vi "From XML.vi"(8 "error in (no error)":errorcluster, 10 "XML String":string, 11 "TOC in":refnum<class "TOC.lvclass">) -> (0 "error out":errorcluster, 3 "TOC out":refnum<class "TOC.lvclass">)   [LabVIEW 2015, in "TOC.lvclass"]
uses:
  TOC.lvclass
  <vilib>/xml/Load XML String.vi
  <vilib>/xml/NI_XML.lvlib
  <resource>/objmgr/DOMUserDefRef.rc
panel:
  out "Node Name":string
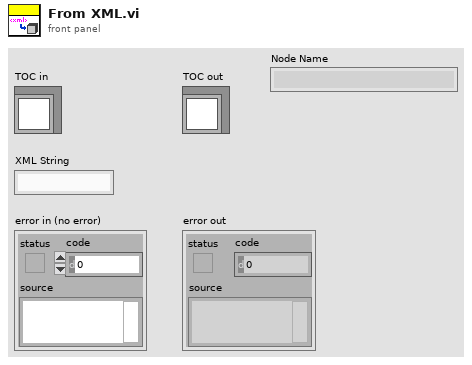
[diagram p1: front panel]
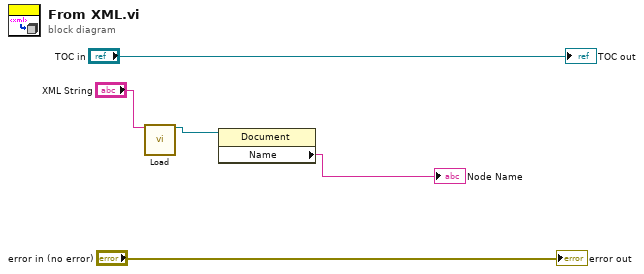
[diagram p0: block diagram]
diagram:
  n1 = call-poly <vilib>:"Load.vi"("XML string"="XML String") -> ("DOM document out"=w2:refnum<k20>)  [unwired: 12 in, 2 out]
  n2 = property class="Document"(reference=w2) -> ("Name"=→"Node Name":string)  [unwired: 1 in, 2 out]
  "error out" <- "error in (no error)"
  "TOC out" <- "TOC in"
